vi "Calculate Feedback.vi"(8 "error in (no error)":errorcluster, 10 "Process variable":dbl, 11 "PID Control in":refnum<class "PID Control.lvclass">) -> (0 "error out":errorcluster, 2 "Feedback":dbl, 3 "PID Control out":refnum<class "PID Control.lvclass">)   [LabVIEW 2016, in "PID Control.lvclass"]
uses:
  PID Control.lvclass
  PID Control.lvclass/PID Control.ctl
  Read PID configuration.vi
  Read dt.vi
  Read Integral accumulator.vi
  Read Set point.vi
  Write Integral accumulator.vi
  Write dt.vi
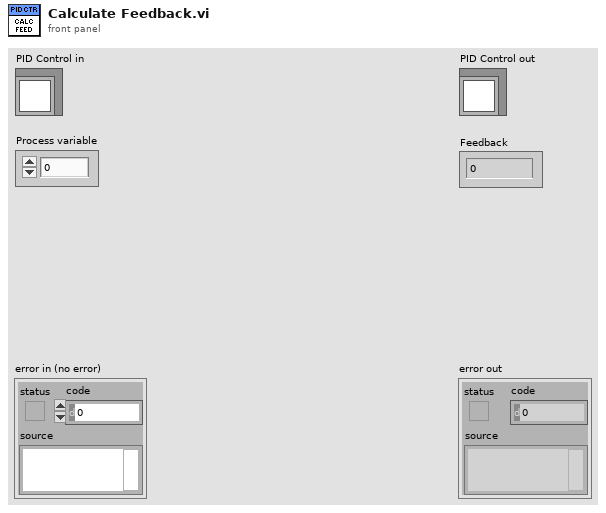
[diagram p1: front panel]
types:
  T1 = typedef "PID Configuration.ctl" = cluster{"Proportional":dbl, "Integral":dbl, "Derivative":dbl}
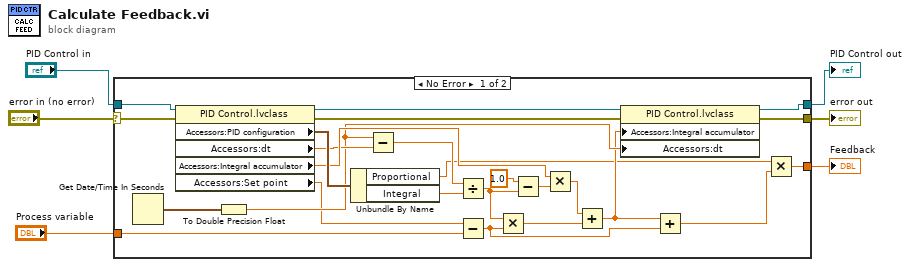
[diagram p0: block diagram]
diagram:
  n1 = case shown="No Error" "error in (no error)" {
    selector: "error in (no error)" -> [w31 w33]
    tunnel: [w17 w33] -> w5
    tunnel: "PID Control in" -> [w30 w32]
    tunnel: "Process variable" -> [w28 _]
    tunnel: [w19 w32] -> w2
    tunnel: [w8 _] -> w1
    frame No Error {
      n2 = Get Date/Time In Seconds() -> (seconds since 1Jan1904=w16:timestamp)
      n3 = property class="PID Control.lvclass"(reference=w30, error in=w31) -> (reference out=w20:refnum<class "PID Control.lvclass">, error out=w18:errorcluster, "Accessors:PID configuration"=w29:T1, "Accessors:dt"=w15:dbl, "Accessors:Integral accumulator"=w25:dbl, "Accessors:Set point"=w7:dbl)
      n4 = To Double Precision Float(number=w16) -> (double precision float=w13:dbl)
      n5 = Unbundle By Name(w29) -> ("Proportional"=w9:dbl, "Integral"=w27:dbl)
      n6 = Subtract(x=w13, y=w15) -> (x-y=w14:dbl)
      n7 = Divide(x=w14, y=w27) -> (x/y=w23:dbl)
      n8 = Subtract(x=w7, y=w28) -> (x-y=w11:dbl)
      n9 = Multiply(x=w23, y=w11) -> (x*y=w21:dbl)
      n10 = Subtract(x=1.0, y=w23) -> (x-y=w24:dbl)
      n11 = Multiply(x=w25, y=w24) -> (x*y=w22:dbl)
      n12 = Add(x=w22, y=w21) -> (x+y=w12:dbl)
      n13 = property class="PID Control.lvclass"(reference=w20, error in=w18, "Accessors:Integral accumulator"=w12, "Accessors:dt"=w13) -> (reference out=w19:refnum<class "PID Control.lvclass">, error out=w17:errorcluster)
      n14 = Add(x=w12, y=w11) -> (x+y=w10:dbl)
      n15 = Multiply(x=w9, y=w10) -> (x*y=w8:dbl)
    }
    frame Error {
    }
  }
  "error out" <- w5
  "PID Control out" <- w2
  "Feedback" <- w1
